vi "FGV_HovaCAL_Interface_SetData.vi"(0 "Set Values Cluster in":T9(array[cluster])=[{"input concentration setpoint"=0.0, "output concentration setpoint"=0.0}, {"input concentration setpoint"=0.0, "output concentration setpoint"=0.0}, {"input concentration setpoint"=0.0, "output concentration setpoint"=0.0}, {"input concentration setpoint"=0.0, "output concentration setpoint"=0.0}, {"input concentration setpoint"=0.0, "output concentration setpoint"=0.0}] {"output concentration setpoint" format="%.2f"; "input concentration setpoint" format="%.2f"}, 1 "PumpModeGeneral-Cluster in":T4 {"dry mode" items=["wet", "dry"]; "control mode" items=["static", "pid"]}, 2 "System Cluster in":T1, 5 "PumpMode-Cluster in":T8(array[cluster]) {"concentratio mode" items=["water", "reagent"]; "Reagent" items=["HCl", "HF", "NH3", "HG", "PPM", "ORGANIC"]}, 7 "total flow setpoint in":dbl, 9 "Temperature":dbl[](array[numeric]) format="%.2f", 11 "Pump Concentrations-Cluster":T5[](array[typedef]), 12 "Aktion":T10, 13 "Limits Cluster in":cluster{"flow":dbl[], "temp":dbl[]}) -> (3 "PumpModeGeneral-Cluster out":T4 {"dry mode" items=["wet", "dry"]; "control mode" items=["static", "pid"]}, 4 "Set Values Cluster out":T9(array[cluster]), 6 "PumpMode-Cluster out":T8(array[cluster]) {"concentratio mode" items=["water", "reagent"]; "Reagent" items=["HCl", "HF", "NH3", "HG", "PPM", "ORGANIC"]}, 8 "total flow setpoint out":dbl, 10 "Temperature out":dbl[](array[numeric]), 14 "Limits Cluster out":cluster{"flow":dbl[], "temp":dbl[]}, 15 "Pump Concentrations-Cluster out":T5[](array[typedef]))   [LabVIEW 2020, in "Linearisierung v2.lvlib" / "Gasteiler.lvlib" / "HovaCAL_Interface.lvlib" / "Kommunikation.lvlib"]
uses:
  Kommunikation.lvlib
  Aktion_FGV_HovaCAL_Interface_SetData.ctl
  Controls/Pump Concentration Mode.ctl
  Controls/Reagent.ctl
  Controls/Pump Concentration.ctl
  Controls/Pump Dry Mode.ctl
  Controls/Pump Control Mode.ctl
  Controls/Info Cluster.ctl
  Aktion FGV Stoerungen sammeln und auswerten.ctl
  LIN ErrorCluster.ctl
  Controls/Controls.lvlib
  Linearisierung v2.lvlib
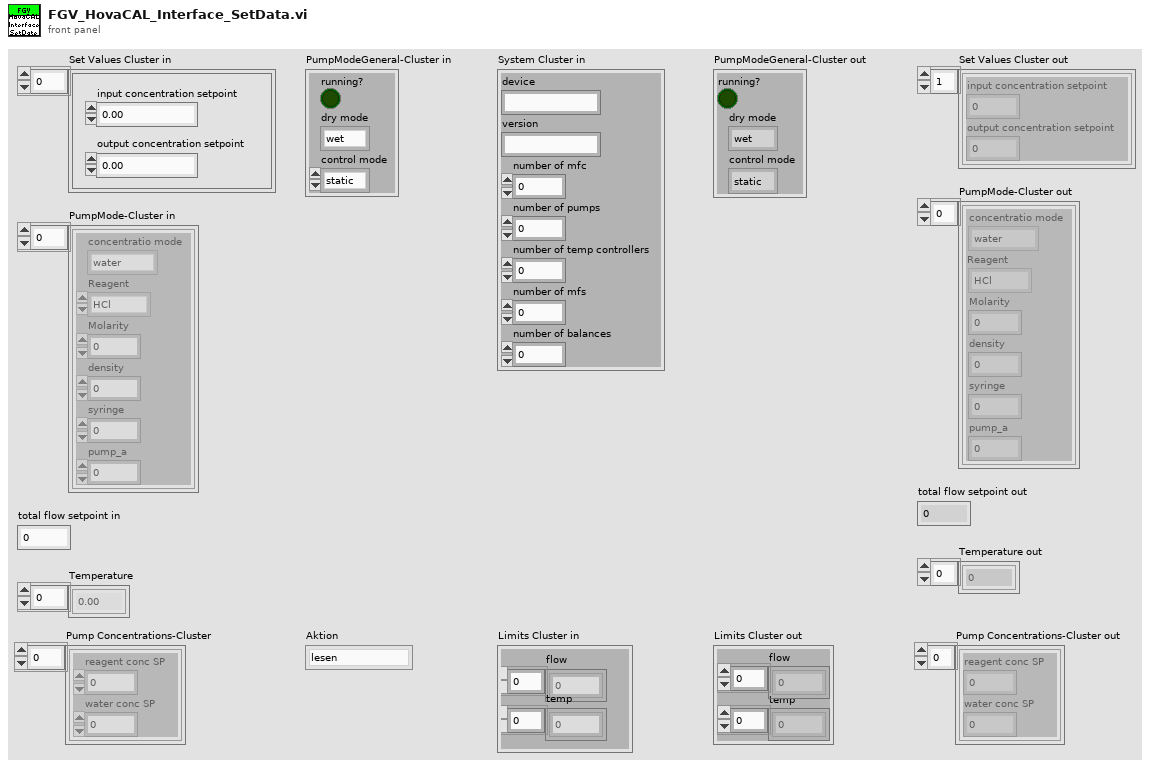
[diagram p1: front panel]
types:
  T1 = typedef "Linearisierung v2.lvlib/Gasteiler.lvlib/HovaCAL_Interface.lvlib/Controls.lvlib/Info Cluster.ctl" = cluster{"device":string, "version":string, "number of mfc":i32, "number of pumps":i32, "number of temp controllers":i32, "number of mfs":i32, "number of balances":i32}
  T2 = typedef "Linearisierung v2.lvlib/Gasteiler.lvlib/HovaCAL_Interface.lvlib/Controls.lvlib/Pump Dry Mode.ctl" = i32
  T3 = typedef "Linearisierung v2.lvlib/Gasteiler.lvlib/HovaCAL_Interface.lvlib/Controls.lvlib/Pump Control Mode.ctl" = u32
  T4 = cluster{"running?":bool, "dry mode":T2, "control mode":T3}
  T5 = typedef "Linearisierung v2.lvlib/Gasteiler.lvlib/HovaCAL_Interface.lvlib/Controls.lvlib/Pump Concentration.ctl" = cluster{"reagent conc SP":dbl, "water conc SP":dbl}
  T6 = typedef "Linearisierung v2.lvlib/Gasteiler.lvlib/HovaCAL_Interface.lvlib/Controls.lvlib/Pump Concentration Mode.ctl" = i32
  T7 = typedef "Linearisierung v2.lvlib/Gasteiler.lvlib/HovaCAL_Interface.lvlib/Controls.lvlib/Reagent.ctl" = i32
  T8 = cluster{"concentratio mode":T6, "Reagent":T7, "Molarity":dbl, "density":dbl, "syringe":dbl, "pump_a":dbl}[]
  T9 = cluster{"input concentration setpoint":dbl, "output concentration setpoint":dbl}[]
  T10 = typedef "Linearisierung v2.lvlib/Gasteiler.lvlib/HovaCAL_Interface.lvlib/Kommunikation.lvlib/Aktion_FGV_HovaCAL_Interface_SetData.ctl" = enum16{"lesen", "Konzentrationen", "Pumpen Parameter", "Pumpe Konzentration", "Pumpe run", "Temperaturen", "Fluss", "Limits", "init"}
  T11 = cluster{"reagent conc SP":dbl, "water conc SP":dbl}
  T12 = cluster{"concentratio mode":T6, "Reagent":T7, "Molarity":dbl, "density":dbl, "syringe":dbl, "pump_a":dbl}
  T13 = cluster{"input concentration setpoint":dbl, "output concentration setpoint":dbl}
  T14 = typedef "Linearisierung v2.lvlib/LIN ErrorCluster.ctl" = cluster{"Störung Kommunikation":bool, "Pressure carrier gas":bool, "Pressure diluted gas":bool, "Outlet Pressure":bool, "SNOX before SAIR":bool, "Störung Gasteiler":bool}
  T15 = typedef "Linearisierung v2.lvlib/Aktion FGV Stoerungen sammeln und auswerten.ctl" = enum16{"init", "lesen", "error", "prüfen", "reset error", "abbrechen", "fortsetzen", "neustart", "Bedientasten reset"}
  T16 = cluster{"reagent conc SP":dbl, "water conc SP":dbl}[]
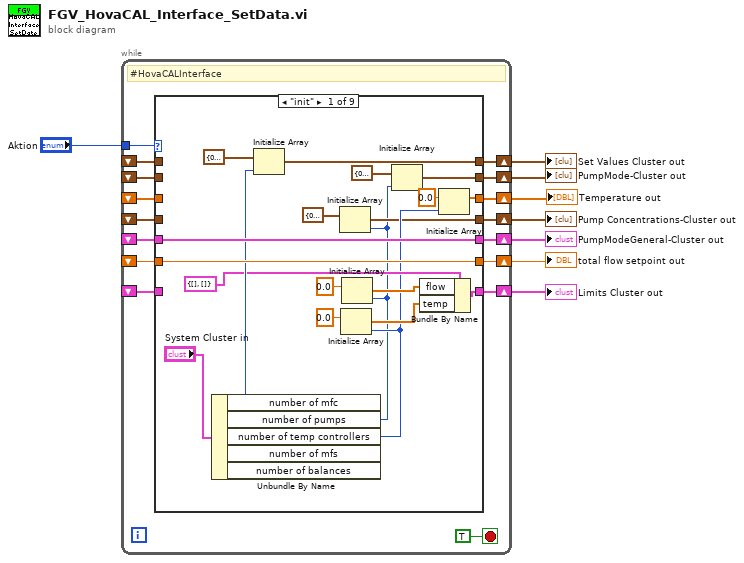
[diagram p0: block diagram]
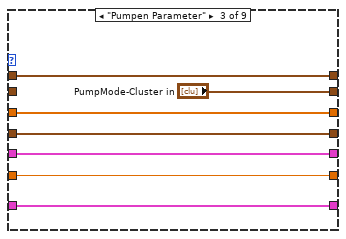
[diagram p3: hidden frame]
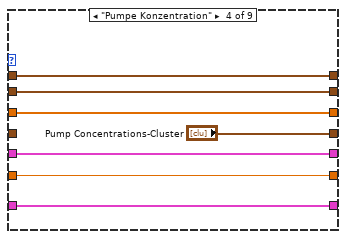
[diagram p4: hidden frame]
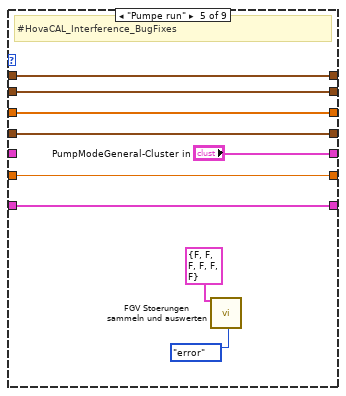
[diagram p5: hidden frame]
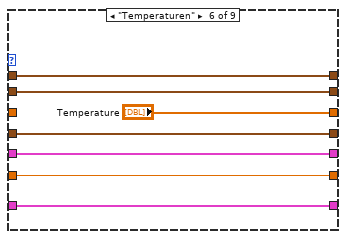
[diagram p6: hidden frame]
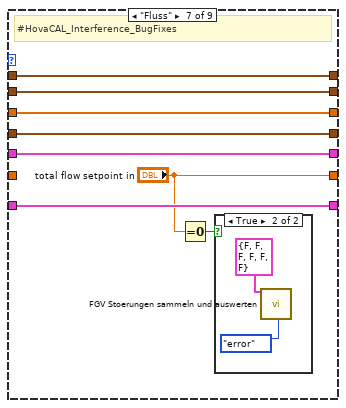
[diagram p7: hidden frame]
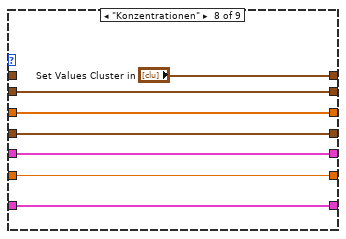
[diagram p9: hidden frame]
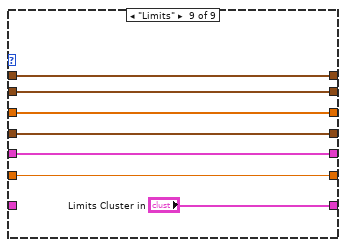
[diagram p10: hidden frame]
diagram:
  n1 = while {
    tunnel: "Aktion" -> [w23]
    shift-right: [w22] -> w7
    shift-left: _ -> [w21]
    shift-right: [w20] -> w6
    shift-left: _ -> [w19]
    shift-right: [w18] -> w5
    shift-left: _ -> [w17]
    shift-right: [w16] -> w4
    shift-left: _ -> [w15]
    shift-right: [w14] -> w3
    shift-left: _ -> [w13]
    shift-right: [w12] -> w2
    shift-left: _ -> [w11]
    shift-right: [w10] -> w1
    shift-left: _ -> [w9]
    stop <- TRUE stop-if-true
    # "#HovaCALInterface"
    n2 = case shown="\"init\"" w23 {
      tunnel: [w39 w51 w58 w65 w74 w81 w89 "Set Values Cluster in" w105] -> w22
      tunnel: w21 -> [_ w51 w58 w65 w74 w81 w89 _ w105]
      tunnel: [w37 w50 "PumpMode-Cluster in" w64 w73 w80 w88 w97 w104] -> w20
      tunnel: w19 -> [_ w50 _ w64 w73 w80 w88 w97 w104]
      tunnel: [w35 w49 w56 w63 w72 "Temperature" w87 w96 w103] -> w18
      tunnel: w17 -> [_ w49 w56 w63 w72 _ w87 w96 w103]
      tunnel: [w26 w48 w55 "Pump Concentrations-Cluster" w71 w78 w86 w95 w102] -> w16
      tunnel: w15 -> [_ w48 w55 _ w71 w78 w86 w95 w102]
      tunnel: [w44 w47 w54 w61 "PumpModeGeneral-Cluster in" w77 w85 w94 w101] -> w14
      tunnel: w13 -> [w44 w47 w54 w61 _ w77 w85 w94 w101]
      tunnel: [w43 w46 w53 w60 w69 w76 "total flow setpoint in" w93 w100] -> w12
      tunnel: w11 -> [w43 w46 w53 w60 w69 w76 _ w93 w100]
      tunnel: [w28 w45 w52 w59 w68 w75 w84 w92 "Limits Cluster in"] -> w10
      tunnel: w9 -> [_ w45 w52 w59 w68 w75 w84 w92 _]
      frame "init" {
        n3 = Unbundle By Name("System Cluster in") -> ("number of mfc"=w41:i32, "number of pumps"=w25:i32, "number of temp controllers"=w29:i32)  [unwired: 2 out]
        n4 = Initialize Array(T13 {"input concentration setpoint"=0.0, "output concentration setpoint"=0.0} ("Set Values Cluster in"), w41) -> (w39:T9)
        n5 = Initialize Array(T11 {"reagent conc SP"=0.0, "water conc SP"=0.0} ("Ausgangs-Cluster"), w25) -> (w26:T16)
        n6 = Initialize Array(0.0 ("temp"), w29) -> (w30:dbl[])
        n7 = Initialize Array(0.0 ("flow"), w25) -> (w31:dbl[])
        n8 = Initialize Array(T12 {"concentratio mode"=0, "Reagent"=0, "Molarity"=0.0, "density"=0.0, "syringe"=0.0, "pump_a"=0.0} ("PumpMode-Cluster in"), w25) -> (w37:T8)
        n9 = Bundle By Name(cluster=cluster{"flow":dbl[], "temp":dbl[]} {"flow"=[], "temp"=[]} ("Limits Cluster in"), "flow"=w31, "temp"=w30) -> (w28:cluster{"flow":dbl[], "temp":dbl[]})
        n10 = Initialize Array(0.0 ("Temperature"), w29) -> (w35:dbl[])
      }
      frame "lesen", Default {
      }
      frame "Pumpen Parameter" {
      }
      frame "Pumpe Konzentration" {
      }
      frame "Pumpe run" {
        # "#HovaCAL_Interference_BugFixes"
        n11 = call "FGV Stoerungen sammeln und auswerten.vi"("Errors"=T14 {"Störung Kommunikation"=FALSE, "Pressure carrier gas"=FALSE, "Pressure diluted gas"=FALSE, "Outlet Pressure"=FALSE, "SNOX before SAIR"=FALSE, "Störung Gasteiler"=FALSE} ("Eingangs-Cluster"), "Aktion"=Aktion_FGV_Stoerungen_sammeln_und_auswerten."error") -> ()  [unwired: 11 in, 7 out]
      }
      frame "Temperaturen" {
      }
      frame "Fluss" {
        # "#HovaCAL_Interference_BugFixes"
        n12 = Equal To 0?(x="total flow setpoint in") -> (x = 0?=w82:bool)
        n13 = case shown="True" w82 {
          frame False {
          }
          frame True {
            n14 = call "FGV Stoerungen sammeln und auswerten.vi"("Errors"=T14 {"Störung Kommunikation"=FALSE, "Pressure carrier gas"=FALSE, "Pressure diluted gas"=FALSE, "Outlet Pressure"=FALSE, "SNOX before SAIR"=FALSE, "Störung Gasteiler"=FALSE} ("Eingangs-Cluster"), "Aktion"=Aktion_FGV_Stoerungen_sammeln_und_auswerten."error") -> ()  [unwired: 11 in, 7 out]
          }
        }
      }
      frame "Konzentrationen" {
      }
      frame "Limits" {
      }
    }
  }
  "Set Values Cluster out" <- w7
  "PumpMode-Cluster out" <- w6
  "Temperature out" <- w5
  "Pump Concentrations-Cluster out" <- w4
  "PumpModeGeneral-Cluster out" <- w3
  "total flow setpoint out" <- w2
  "Limits Cluster out" <- w1
